vi "testParametrieren.vi"() -> ()   [LabVIEW 2013]
uses:
  <vilib>/CANopenLib/CANOPEN.llb/CANopen BaudRate.ctl
  <vilib>/CANopenLib/CANOPEN.llb/CANopen Interface Create.vi
panel:
  in  "baud rate":T1 items=["1 Mbit/s"=0, "800 kbit/s"=1, "500 kbit/s"=2, "250 kbit/s"=3, "125 kbit/s"=4, "50 kbit/s"=6, "20 kbit/s"=7, "10 kbit/s"=8]
  out "SR Status":u16
  out "error out":errorcluster caption="Fehler (Ausgang)"
  in  "error in (no error)":errorcluster caption="Fehler (Eingang, kein Fehler)"
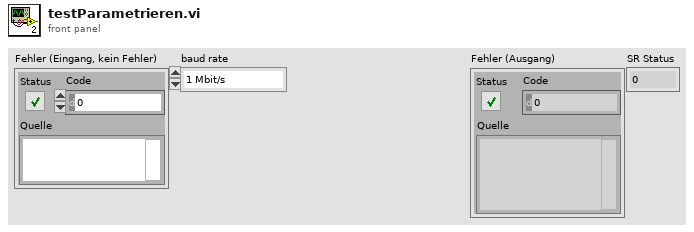
[diagram p1: front panel]
types:
  T1 = typedef "CANopen BaudRate.ctl" = u32
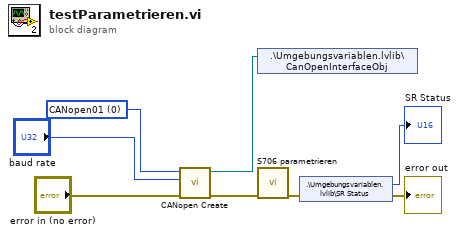
[diagram p0: block diagram]
diagram:
  w5 = u32 0 items=["CANopen01", "CANopen02", "CANopen03", "CANopen04", "CANopen05", "CANopen06", "CANopen07", "CANopen08", "CANopen09", "CANopen10", "CANopen11", "CANopen12", "CANopen13", "CANopen14", "CANopen15", "CANopen16", "CANopen17", "CANopen18", "CANopen19", "CANopen20", "CANopen21", "CANopen22", "CANopen23", "CANopen24", "CANopen25", "CANopen26", "CANopen27", "CANopen28", "CANopen29", "CANopen30", "CANopen31", "CANopen32"] ("interface name")
  n1 = call-poly <vilib>:"CANopen Create.vi"("error in (no error)"="error in (no error)", "baud rate"="baud rate", "interface name"=w5) -> ("error out"=w7:errorcluster, "interface object out"=w8:refnum<k20>)  [unwired: 7 in]
  n2 = shared-variable ".\\Umgebungsvariablen.lvlib\\CanOpenInterfaceObj"(w8) -> ()  [unwired: 1 in, 1 out]
  n3 = call "S706 parametrieren.vi"("error in (no error)"=w7) -> ("error out"=w4:errorcluster)  [unwired: 10 in]
  n4 = shared-variable ".\\Umgebungsvariablen.lvlib\\SR Status"(error in=w4) -> (→"SR Status":u16, error out=→"error out":errorcluster)
